vi "BusEvents.vi"(0 "EventArray":variant[](array[variant]), 7 "Error in":errorcluster[](array[cluster]), 10 "ModuleList":string[](array[string])) -> (19 "output cluster":T8, 20 "SyncEvts":T3, 21 "FGenEvts":T2, 22 "DigitizerEvts":T1, 23 "AnalysisBroadcastEvents":T4, 24 "SensorBdcstEvents":T5, 25 "ScopeBdcstEvents":T6, 26 "clAcPwrEvents":T7, 27 "Error out":errorcluster[](array[cluster]))   [LabVIEW 2018, in "Bus.lvclass"]
uses:
  Bus.lvclass
  Digitizer/DigitizerModule/Protected/Broadcasts/clBroadcastEvents.ctl
  Digitizer/DigitizerModule/Protected/clEventType.ctl
  FGen/FgenModule/Protected/Broadcasts/clBroadcastEvents.ctl
  FGen/FgenModule/Protected/clEventType.ctl
  Sync/SyncModule/Protected/Broadcasts/clBroadcastEvents.ctl
  Sync/SyncModule/Protected/clEventType.ctl
  Analysis/AnalysisModule/Protected/Broadcasts/clBroadcastEvents.ctl
  Analysis/AnalysisModule/Protected/clEventType.ctl
  Sensor/SensorModule/Protected/Broadcasts/clBroadcastEvents.ctl
  Sensor/SensorModule/Protected/clEventType.ctl
  Scope/ScopeModule/Protected/Broadcasts/clBroadcastEvents.ctl
  Scope/ScopeModule/Protected/clEventType.ctl
  AcPwr/AcPwrModule/Protected/Broadcasts/clBroadcastEvents.ctl
  AcPwr/AcPwrModule/Protected/clEventType.ctl
  <vilib>/Utility/error.llb/Error Cluster From Error Code.vi
  <vilib>/ErrorRing/Error Ring.xnode
  Digitizer/DigitizerModule/DigitizerModule.lvlib
  FGen/FgenModule/FgenModule.lvlib
  Sync/SyncModule/SyncModule.lvlib
  <userlib>/NIST/NISTErrorLib/NISTErrorLib.lvlib
  Analysis/AnalysisModule/AnalysisModule.lvlib
  Sensor/SensorModule/SensorModule.lvlib
  Scope/ScopeModule/ScopeModule.lvlib
  AcPwr/AcPwrModule/AcPwrModule.lvlib
panel:
  # "If you want to add other Broadcast Events, open this typedef, copy an existing event and rename it to your event name.\n\nNext create an \"arg\" typedef for the  data and put it into PublicAPI/Arguments/Broadcasts\n\nAfter that, you will need to create a new roadcast vi in Protected/Broadcast.  Look at DidInit.vi or the reportError.vi as examples."
  # "If you want to add other Broadcast Events, open this typedef, copy an existing event and rename it to your event name.\n\nNext create an \"arg\" typedef for the  data and put it into PublicAPI/Arguments/Broadcasts\n\nAfter that, you will need to create a new roadcast vi in Protected/Broadcast.  Look at DidInit.vi or the reportError.vi as examples."
  # "If you want to add other Broadcast Events, open this typedef, copy an existing event and rename it to your event name.\n\nNext create an \"arg\" typedef for the  data and put it into PublicAPI/Arguments/Broadcasts\n\nAfter that, you will need to create a new roadcast vi in Protected/Broadcast.  Look at DidInit.vi or the reportError.vi as examples."
  # "If you want to add other Broadcast Events, open this typedef, copy an existing event and rename it to your event name.\n\nNext create an \"arg\" typedef for the  data and put it into PublicAPI/Arguments/Broadcasts\n\nAfter that, you will need to create a new roadcast vi in Protected/Broadcast.  Look at DidInit.vi or the reportError.vi as examples."
  # "If you want to add other Broadcast Events, open this typedef, copy an existing event and rename it to your event name.\n\nNext create an \"arg\" typedef for the  data and put it into PublicAPI/Arguments/Broadcasts\n\nAfter that, you will need to create a new roadcast vi in Protected/Broadcast.  Look at DidInit.vi or the reportError.vi as examples."
  # "If you want to add other Broadcast Events, open this typedef, copy an existing event and rename it to your event name.\n\nNext create an \"arg\" typedef for the  data and put it into PublicAPI/Arguments/Broadcasts\n\nAfter that, you will need to create a new roadcast vi in Protected/Broadcast.  Look at DidInit.vi or the reportError.vi as examples."
  # "If you want to add other Broadcast Events, open this typedef, copy an existing event and rename it to your event name.\n\nNext create an \"arg\" typedef for the  data and put it into PublicAPI/Arguments/Broadcasts\n\nAfter that, you will need to create a new roadcast vi in Protected/Broadcast.  Look at DidInit.vi or the reportError.vi as examples."
  # "If you want to add other Broadcast Events, open this typedef, copy an existing event and rename it to your event name.\n\nNext create an \"arg\" typedef for the  data and put it into PublicAPI/Arguments/Broadcasts\n\nAfter that, you will need to create a new roadcast vi in Protected/Broadcast.  Look at DidInit.vi or the reportError.vi as examples."
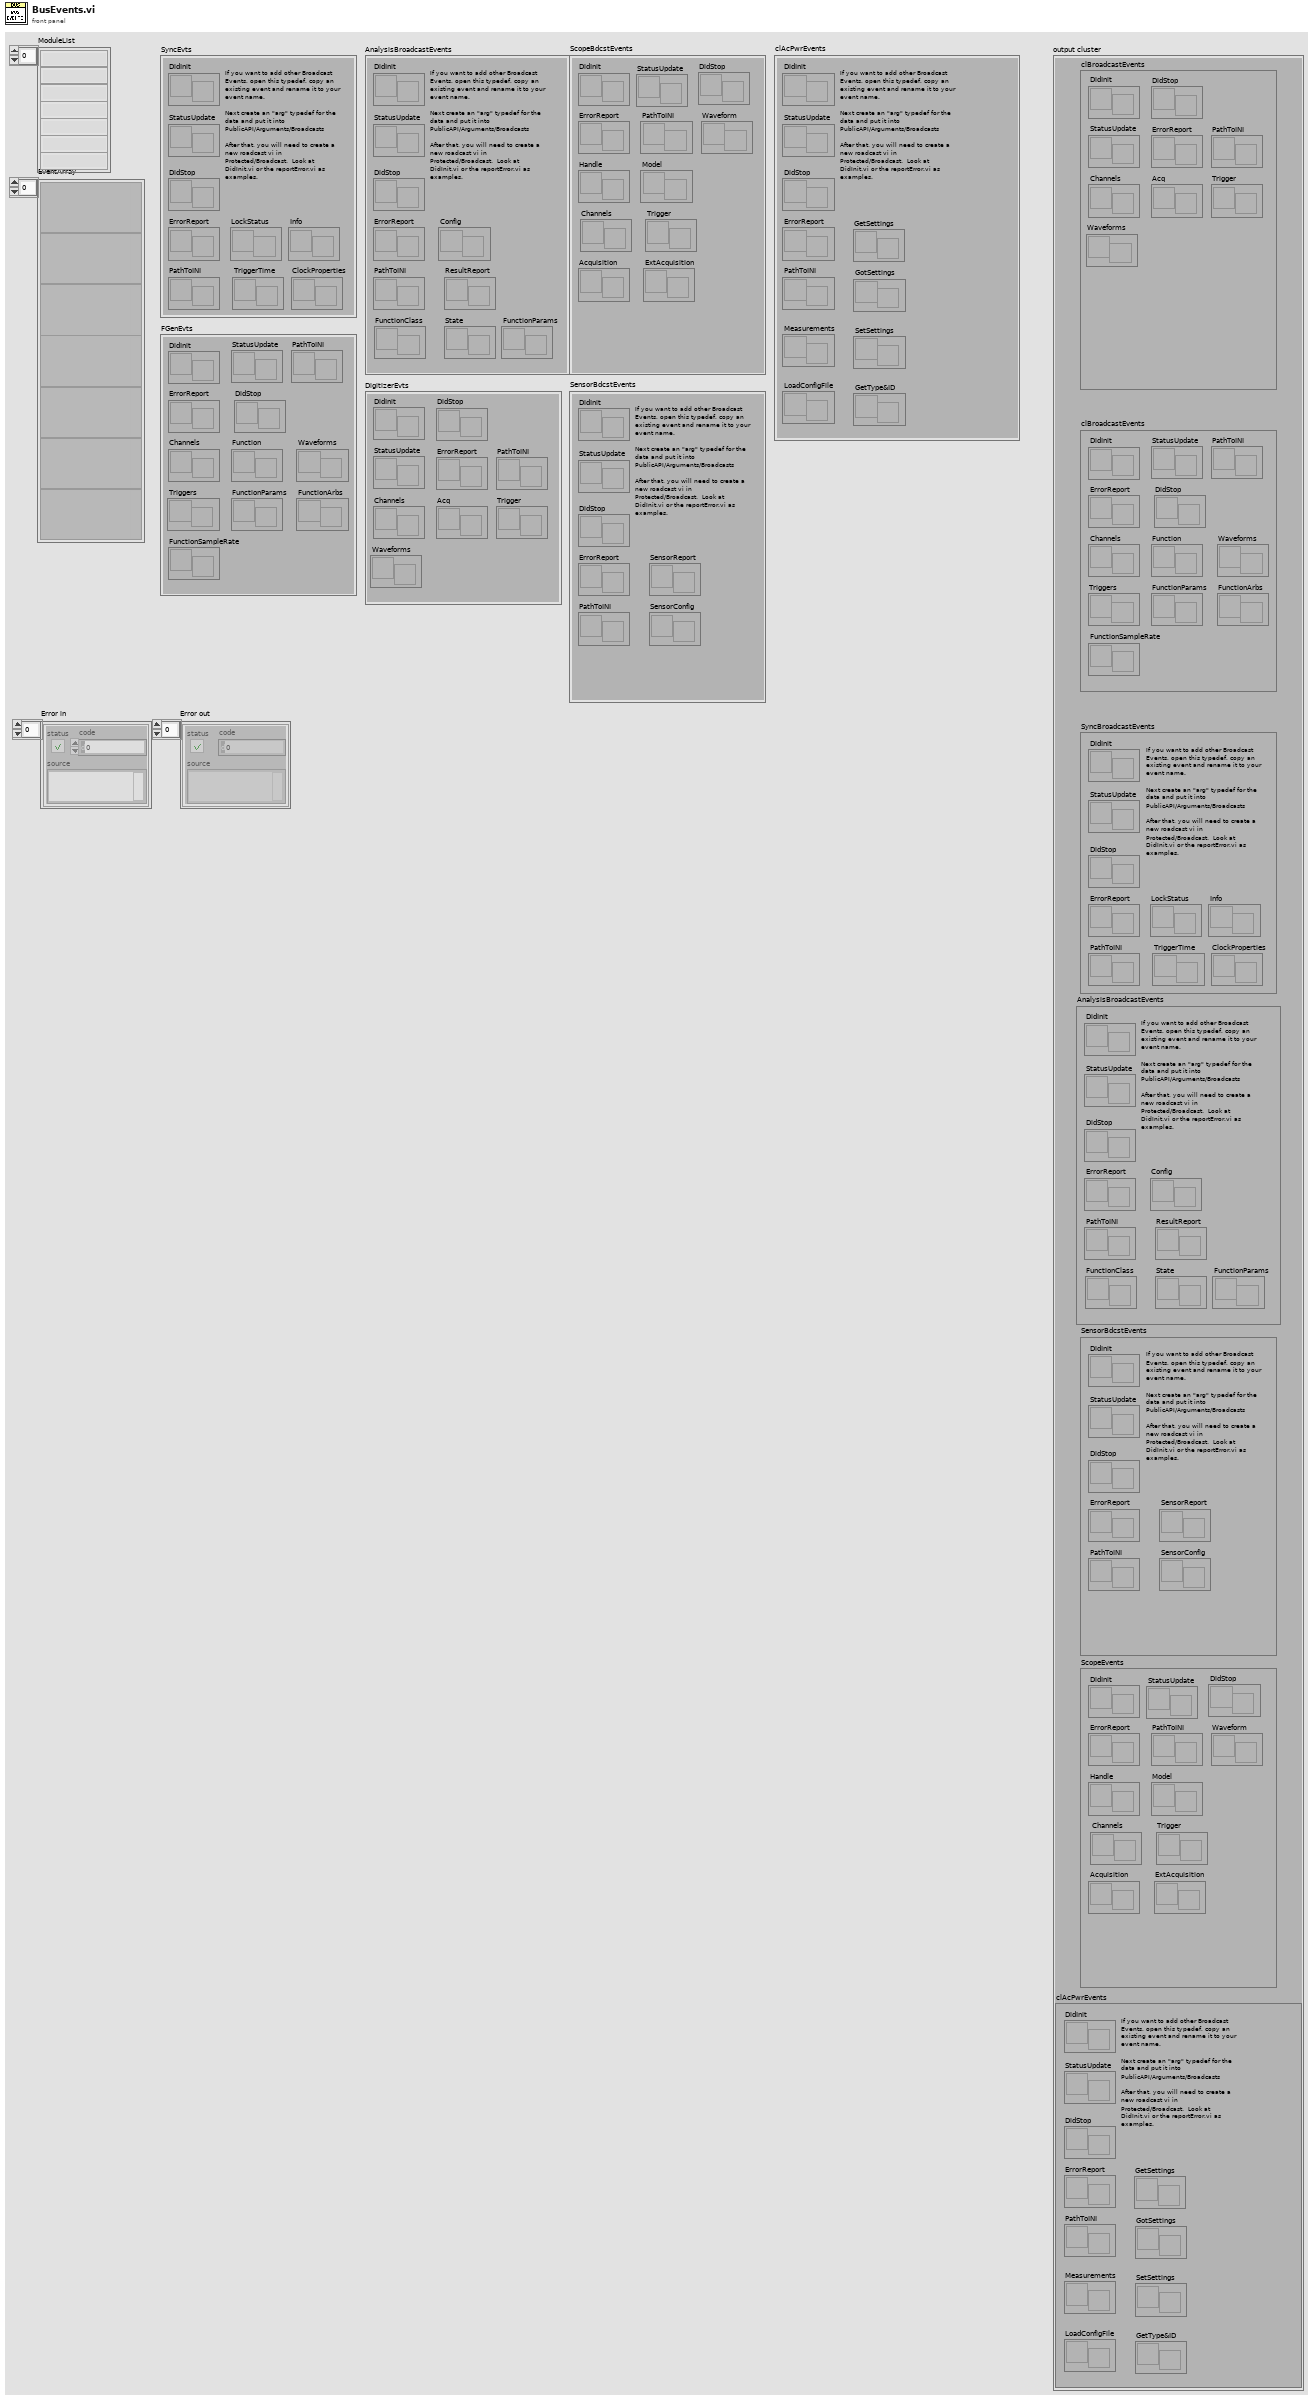
[diagram p1: front panel]
types:
  T1 = typedef "DigitizerModule.lvlib/clBroadcastEvents.ctl" = cluster{"DidInit":refnum<user-event>, "StatusUpdate":refnum<user-event>, "ErrorReport":refnum<user-event>, "DidStop":refnum<user-event>, "PathToINI":refnum<user-event>, "Channels":refnum<user-event>, "Acq":refnum<user-event>, "Trigger":refnum<user-event>, "Waveforms":refnum<user-event>}
  T2 = typedef "FgenModule.lvlib/clBroadcastEvents.ctl" = cluster{"DidInit":refnum<user-event>, "StatusUpdate":refnum<user-event>, "ErrorReport":refnum<user-event>, "DidStop":refnum<user-event>, "PathToINI":refnum<user-event>, "Channels":refnum<user-event>, "Function":refnum<user-event>, "Waveforms":refnum<user-event>, "Triggers":refnum<user-event>, "FunctionParams":refnum<user-event>, "FunctionArbs":refnum<user-event>, "FunctionSampleRate":refnum<user-event>}
  T3 = typedef "SyncModule.lvlib/clBroadcastEvents.ctl" = cluster{"DidInit":refnum<user-event>, "StatusUpdate":refnum<user-event>, "ErrorReport":refnum<user-event>, "DidStop":refnum<user-event>, "PathToINI":refnum<user-event>, "TriggerTime":refnum<user-event>, "LockStatus":refnum<user-event>, "Info":refnum<user-event>, "ClockProperties":refnum<user-event>}
  T4 = typedef "AnalysisModule.lvlib/clBroadcastEvents.ctl" = cluster{"DidInit":refnum<user-event>, "StatusUpdate":refnum<user-event>, "ErrorReport":refnum<user-event>, "DidStop":refnum<user-event>, "PathToINI":refnum<user-event>, "Config":refnum<user-event>, "ResultReport":refnum<user-event>, "FunctionClass":refnum<user-event>, "State":refnum<user-event>, "FunctionParams":refnum<user-event>}
  T5 = typedef "SensorModule.lvlib/clBroadcastEvents.ctl" = cluster{"DidInit":refnum<user-event>, "StatusUpdate":refnum<user-event>, "ErrorReport":refnum<user-event>, "DidStop":refnum<user-event>, "PathToINI":refnum<user-event>, "SensorReport":refnum<user-event>, "SensorConfig":refnum<user-event>}
  T6 = typedef "ScopeModule.lvlib/clBroadcastEvents.ctl" = cluster{"DidInit":refnum<user-event>, "StatusUpdate":refnum<user-event>, "ErrorReport":refnum<user-event>, "DidStop":refnum<user-event>, "PathToINI":refnum<user-event>, "Handle":refnum<user-event>, "Model":refnum<user-event>, "Channels":refnum<user-event>, "Acquisition":refnum<user-event>, "Trigger":refnum<user-event>, "ExtAcquisition":refnum<user-event>, "Waveform":refnum<user-event>}
  T7 = typedef "AcPwrModule.lvlib/clBroadcastEvents.ctl" = cluster{"DidInit":refnum<user-event>, "StatusUpdate":refnum<user-event>, "ErrorReport":refnum<user-event>, "DidStop":refnum<user-event>, "PathToINI":refnum<user-event>, "Measurements":refnum<user-event>, "LoadConfigFile":refnum<user-event>, "GetSettings":refnum<user-event>, "SetSettings":refnum<user-event>, "GetType&ID":refnum<user-event>, "GotSettings":refnum<user-event>}
  T8 = cluster{"clBroadcastEvents":T1, "clBroadcastEvents":T2, "SyncBroadcastEvents":T3, "AnalysisBroadcastEvents":T4, "SensorBdcstEvents":T5, "ScopeEvents":T6, "clAcPwrEvents":T7}
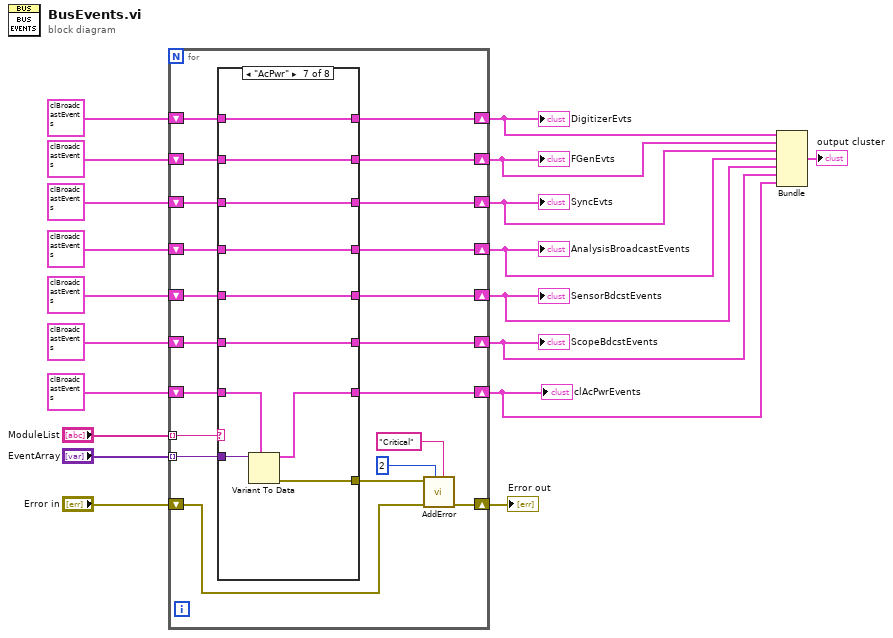
[diagram p0: block diagram]
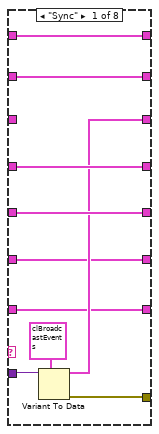
[diagram p2: hidden frame]
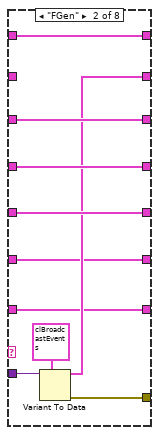
[diagram p3: hidden frame]
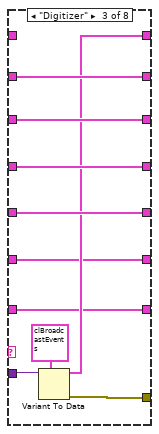
[diagram p4: hidden frame]
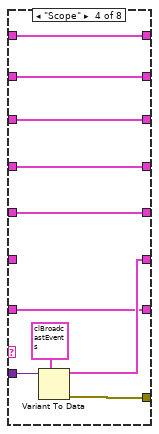
[diagram p5: hidden frame]
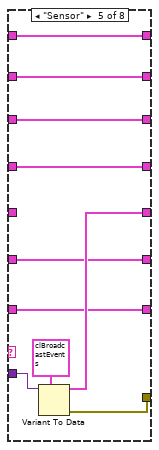
[diagram p6: hidden frame]
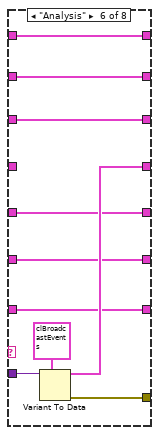
[diagram p7: hidden frame]
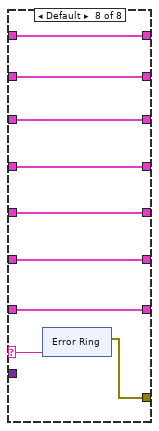
[diagram p8: hidden frame]
diagram:
  n1 = for {
    tunnel: "ModuleList" -> [w36] mode=indexing
    tunnel: "EventArray" -> [w35] mode=indexing
    shift-right: [w38] -> w14
    shift-left: "Error in" -> [w37]
    shift-right: [w32] -> w4
    shift-left: T1 {"DidInit"=refnum, "StatusUpdate"=refnum, "ErrorReport"=refnum, "DidStop"=refnum, "PathToINI"=refnum, "Channels"=refnum, "Acq"=refnum, "Trigger"=refnum, "Waveforms"=refnum} ("clBroadcastEvents") -> [w33]
    shift-right: [w28] -> w8
    shift-left: T3 {"DidInit"=refnum, "StatusUpdate"=refnum, "ErrorReport"=refnum, "DidStop"=refnum, "PathToINI"=refnum, "TriggerTime"=refnum, "LockStatus"=refnum, "Info"=refnum, "ClockProperties"=refnum} ("SyncBroadcastEvents") -> [w30]
    shift-right: [w29] -> w2
    shift-left: T2 {"DidInit"=refnum, "StatusUpdate"=refnum, "ErrorReport"=refnum, "DidStop"=refnum, "PathToINI"=refnum, "Channels"=refnum, "Function"=refnum, "Waveforms"=refnum, "Triggers"=refnum, "FunctionParams"=refnum, "FunctionArbs"=refnum, "FunctionSampleRate"=refnum} ("clBroadcastEvents") -> [w31]
    shift-right: [w26] -> w7
    shift-left: T4 {"DidInit"=refnum, "StatusUpdate"=refnum, "ErrorReport"=refnum, "DidStop"=refnum, "PathToINI"=refnum, "Config"=refnum, "ResultReport"=refnum, "FunctionClass"=refnum, "State"=refnum, "FunctionParams"=refnum} ("AnalysisBroadcastEvents") -> [w27]
    shift-right: [w24] -> w6
    shift-left: T5 {"DidInit"=refnum, "StatusUpdate"=refnum, "ErrorReport"=refnum, "DidStop"=refnum, "PathToINI"=refnum, "SensorReport"=refnum, "SensorConfig"=refnum} ("SensorBdcstEvents") -> [w25]
    shift-right: [w22] -> w5
    shift-left: T6 {"DidInit"=refnum, "StatusUpdate"=refnum, "ErrorReport"=refnum, "DidStop"=refnum, "PathToINI"=refnum, "Handle"=refnum, "Model"=refnum, "Channels"=refnum, "Acquisition"=refnum, "Trigger"=refnum, "ExtAcquisition"=refnum, "Waveform"=refnum} ("ScopeEvents") -> [w23]
    shift-right: [w20] -> w9
    shift-left: T7 {"DidInit"=refnum, "StatusUpdate"=refnum, "ErrorReport"=refnum, "DidStop"=refnum, "PathToINI"=refnum, "Measurements"=refnum, "LoadConfigFile"=refnum, "GetSettings"=refnum, "SetSettings"=refnum, "GetType&ID"=refnum, "GotSettings"=refnum} ("clAcPwrEvents") -> [w21]
    n2 = case shown="\"AcPwr\"" w36 {
      selector: w36 -> [_ _ _ _ _ _ _ w116]
      tunnel: w35 -> [w49 w60 w66 w77 w87 w100 w110 _]
      tunnel: [w48 w59 w70 w80 w90 w99 w109 w115] -> w34
      tunnel: w33 -> [w46 w57 _ w72 w85 w96 w108 w119]
      tunnel: [w46 w57 w63 w72 w85 w96 w108 w119] -> w32
      tunnel: w31 -> [w47 _ w68 w79 w89 w95 w107 w118]
      tunnel: [w47 w53 w68 w79 w89 w95 w107 w118] -> w29
      tunnel: w30 -> [_ w56 w67 w78 w88 w94 w106 w117]
      tunnel: [w43 w56 w67 w78 w88 w94 w106 w117] -> w28
      tunnel: [w45 w55 w65 w76 w86 w97 w103 w114] -> w26
      tunnel: w27 -> [w45 w55 w65 w76 w86 _ w103 w114]
      tunnel: [w44 w54 w64 w75 w83 w93 w105 w113] -> w24
      tunnel: w25 -> [w44 w54 w64 w75 _ w93 w105 w113]
      tunnel: w23 -> [w42 w52 w62 _ w82 w92 w104 w112]
      tunnel: [w42 w52 w62 w73 w82 w92 w104 w112] -> w22
      tunnel: w21 -> [w41 w51 w61 w71 w81 w91 w102 w111]
      tunnel: [w41 w51 w61 w71 w81 w91 w101 w111] -> w20
      frame "Sync" {
        n3 = Variant To Data(type=T3 {"DidInit"=refnum, "StatusUpdate"=refnum, "ErrorReport"=refnum, "DidStop"=refnum, "PathToINI"=refnum, "TriggerTime"=refnum, "LockStatus"=refnum, "Info"=refnum, "ClockProperties"=refnum} ("SyncBroadcastEvents"), Variant=w49) -> (data=w43:T3, error out=w48:errorcluster)  [unwired: 1 in]
      }
      frame "FGen" {
        n4 = Variant To Data(type=T2 {"DidInit"=refnum, "StatusUpdate"=refnum, "ErrorReport"=refnum, "DidStop"=refnum, "PathToINI"=refnum, "Channels"=refnum, "Function"=refnum, "Waveforms"=refnum, "Triggers"=refnum, "FunctionParams"=refnum, "FunctionArbs"=refnum, "FunctionSampleRate"=refnum} ("clBroadcastEvents"), Variant=w60) -> (data=w53:T2, error out=w59:errorcluster)  [unwired: 1 in]
      }
      frame "Digitizer" {
        n5 = Variant To Data(type=T1 {"DidInit"=refnum, "StatusUpdate"=refnum, "ErrorReport"=refnum, "DidStop"=refnum, "PathToINI"=refnum, "Channels"=refnum, "Acq"=refnum, "Trigger"=refnum, "Waveforms"=refnum} ("clBroadcastEvents"), Variant=w66) -> (data=w63:T1, error out=w70:errorcluster)  [unwired: 1 in]
      }
      frame "Scope" {
        n6 = Variant To Data(type=T6 {"DidInit"=refnum, "StatusUpdate"=refnum, "ErrorReport"=refnum, "DidStop"=refnum, "PathToINI"=refnum, "Handle"=refnum, "Model"=refnum, "Channels"=refnum, "Acquisition"=refnum, "Trigger"=refnum, "ExtAcquisition"=refnum, "Waveform"=refnum} ("ScopeEvents"), Variant=w77) -> (data=w73:T6, error out=w80:errorcluster)  [unwired: 1 in]
      }
      frame "Sensor" {
        n7 = Variant To Data(type=T5 {"DidInit"=refnum, "StatusUpdate"=refnum, "ErrorReport"=refnum, "DidStop"=refnum, "PathToINI"=refnum, "SensorReport"=refnum, "SensorConfig"=refnum} ("SensorBdcstEvents"), Variant=w87) -> (data=w83:T5, error out=w90:errorcluster)  [unwired: 1 in]
      }
      frame "Analysis" {
        n8 = Variant To Data(type=T4 {"DidInit"=refnum, "StatusUpdate"=refnum, "ErrorReport"=refnum, "DidStop"=refnum, "PathToINI"=refnum, "Config"=refnum, "ResultReport"=refnum, "FunctionClass"=refnum, "State"=refnum, "FunctionParams"=refnum} ("AnalysisBroadcastEvents"), Variant=w100) -> (data=w97:T4, error out=w99:errorcluster)  [unwired: 1 in]
      }
      frame "AcPwr" {
        n9 = Variant To Data(type=w102, Variant=w110) -> (data=w101:T7, error out=w109:errorcluster)  [unwired: 1 in]
      }
      frame Default {
        n10 = xnode "Error Ring"("parameter 0"=w116) -> ("error out"=w115:errorcluster)
      }
    }
    n11 = call <userlib>:"AddError.vi"("Severity"="Critical", "Priority"=u8 2, "ErrorArray"=w37, "error in (no error)"=w34) -> ("ErrorArray"=w38:errorcluster[])  [unwired: 6 in, 1 out]
  }
  "Error out" <- w14
  "DigitizerEvts" <- w4
  "FGenEvts" <- w2
  "SyncEvts" <- w8
  "AnalysisBroadcastEvents" <- w7
  "SensorBdcstEvents" <- w6
  "ScopeBdcstEvents" <- w5
  "clAcPwrEvents" <- w9
  n12 = Bundle("clBroadcastEvents"=w4, "clBroadcastEvents"=w2, "SyncBroadcastEvents"=w8, "AnalysisBroadcastEvents"=w7, "SensorBdcstEvents"=w6, "ScopeEvents"=w5, "clAcPwrEvents"=w9) -> (→"output cluster":T8)  [unwired: 1 in]
